vi "Create Framework.vi"(8 "error in (no error)":errorcluster, 11 "Application Data in":T1={"Item Tree Control"=refnum, "Top-Level VI"=refnum, "menu reference"=refnum, "queue"=refnum, "Stop Pointer"=refnum, "Buffer Variant"=variant, "server ID"=refnum, "framework tag"="", "Values"=refnum, "Hex"=refnum, "ASCII"=refnum, "lines visible"=0, "values padding"=0, "current buffer data"={"decimation"=0, "avg bandwidth"=0.0, "channels"=[], "byte order"=enum."little-endian", "buffer descriptor"={"buffer type"=enum."Engine", "plugin id"=0, "group id"=0, "transfer id"=0, "offset"=0, "length"=0}, "values channels"={"index"=0, "count"=0, "engine offset"=0}, "select start offset"=18446744073709551615, "select end offset"=0, "channel index"=-1}, "Framework Configuration"=refnum} {"current buffer data"."channels"."configuration"."string offset" format="%d bytes"; "current buffer data"."avg bandwidth" format="%.0g bytes"}) -> (0 "error out":errorcluster, 2 "framework tag":string, 3 "Application Data Out":T1={"Item Tree Control"=refnum, "Top-Level VI"=refnum, "menu reference"=refnum, "queue"=refnum, "Stop Pointer"=refnum, "Buffer Variant"=variant, "server ID"=refnum, "framework tag"="", "Values"=refnum, "Hex"=refnum, "ASCII"=refnum, "lines visible"=0, "values padding"=0, "current buffer data"={"decimation"=0, "avg bandwidth"=0.0, "channels"=[], "byte order"=enum."little-endian", "buffer descriptor"={"buffer type"=enum."Engine", "plugin id"=0, "group id"=0, "transfer id"=0, "offset"=0, "length"=0}, "values channels"={"index"=0, "count"=0, "engine offset"=0}, "select start offset"=18446744073709551615, "select end offset"=0, "channel index"=-1}, "Framework Configuration"=refnum} {"current buffer data"."channels"."configuration"."string offset" format="%d bytes"; "current buffer data"."avg bandwidth" format="%.0g bytes"})   [LabVIEW 2019, in "DSF Core.lvlib"]
uses:
  DSF Core.lvlib
  Main VI/Application Data.ctl
  <vilib>/NI/Memory Manager/Classes/Pointer/Pointer.lvclass
  Classes/Configuration/Core/Framework/Framework Configuration.lvclass
  Buffer Reader/Queue Data.ctl
  Buffer Reader/Buffer Data.ctl
  Classes/Configuration/Core/Transfer/Channel Configuration.ctl
  Typedefs/Core Channel Configuration.ctl
  Typedefs/DSF Data Type.ctl
  Typedefs/DSF Settings Info.ctl
  Typedefs/DSF Byte Order.ctl
  Classes/Thread/Data Server/DSF Buffer Subset Descriptor.ctl
  Typedefs/DSF Buffer Type.ctl
  Main VI/Values Channels.ctl
  ID to Tree Items/Tree Item Type.ctl
  Classes/Configuration/Core/Channel/Channel Configuration.lvclass
  Classes/Configuration/Core/Transfer/Transfer Configuration.lvclass
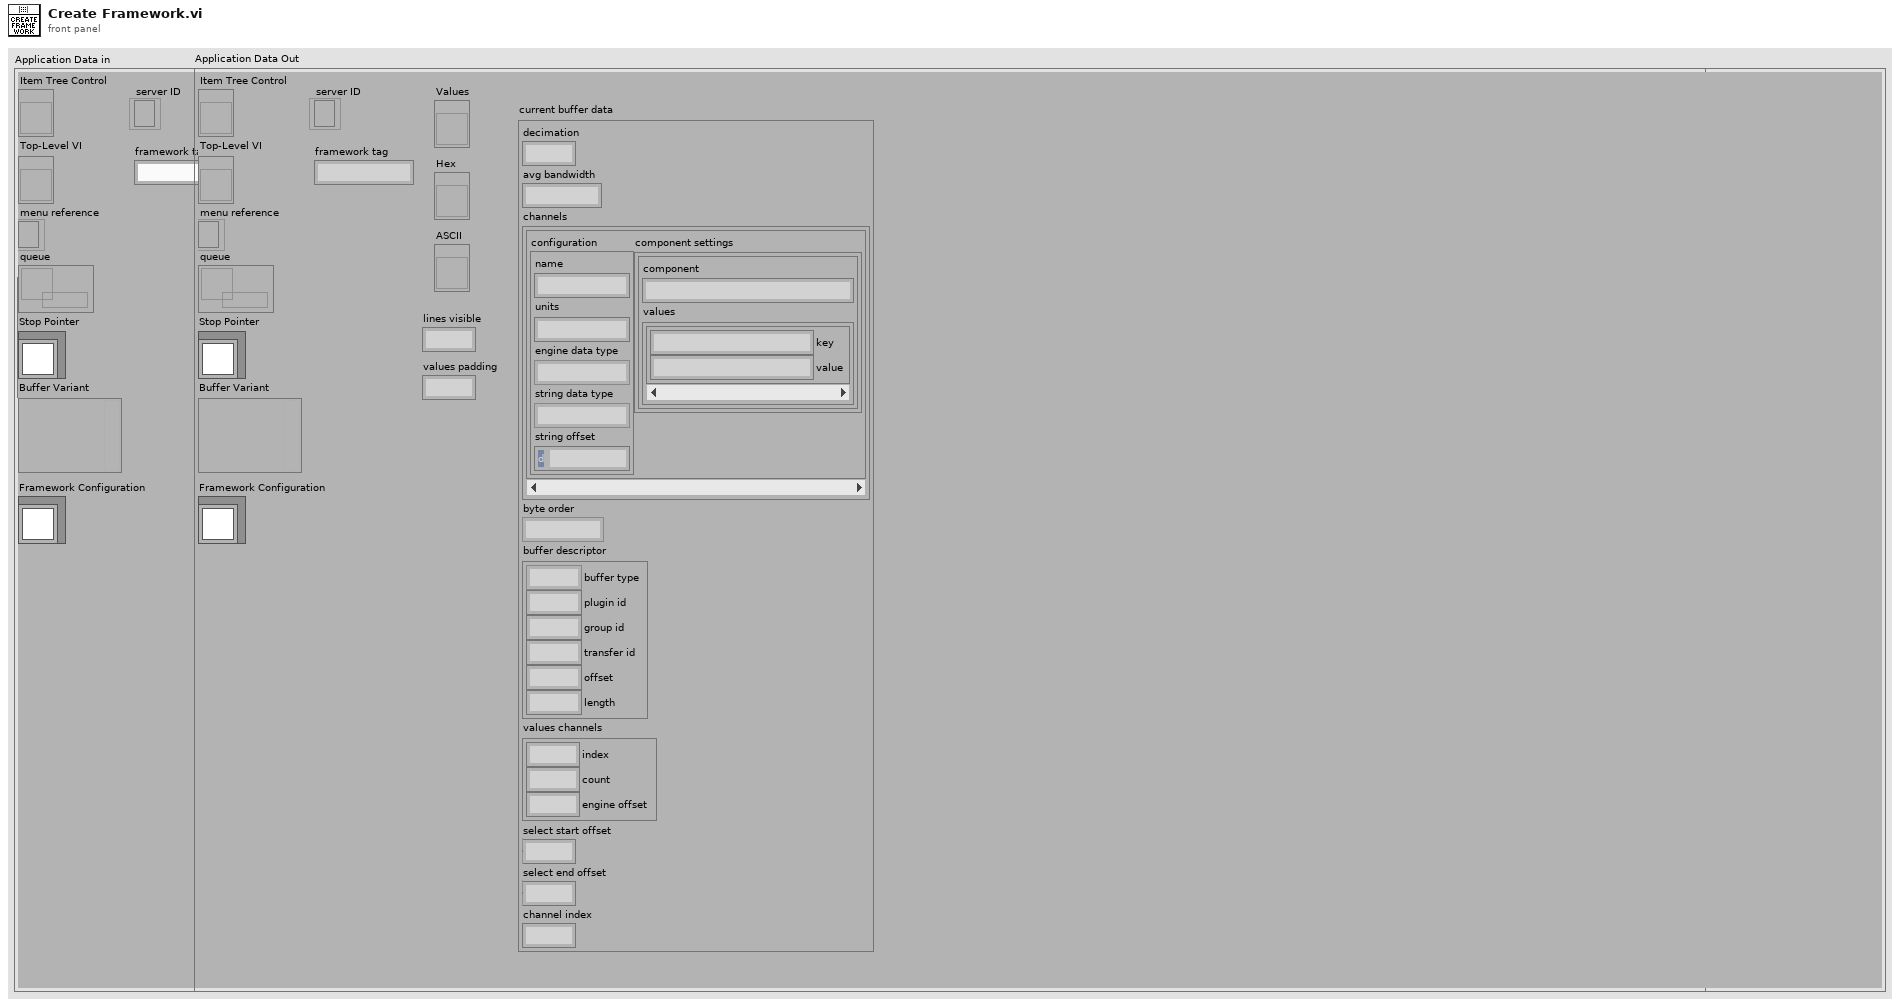
[diagram p1: front panel]
types:
  T1 = typedef "DSF Core.lvlib/Application Data.ctl" = cluster{"Item Tree Control":refnum<vi>, "Top-Level VI":refnum<vi>, "menu reference":refnum<k9>, "queue":refnum<queue>, "Stop Pointer":refnum<class "Pointer.lvclass">, "Buffer Variant":variant, "server ID":refnum<k5>, "framework tag":string, "Values":refnum<vi>, "Hex":refnum<vi>, "ASCII":refnum<vi>, "lines visible":i32, "values padding":i32, "current buffer data":T2, "Framework Configuration":refnum<class "Framework Configuration.lvclass">}
  T2 = typedef "DSF Core.lvlib/Buffer Data.ctl" = cluster{"decimation":u64, "avg bandwidth":dbl, "channels":T3[], "byte order":T7, "buffer descriptor":T8, "values channels":T10, "select start offset":u64, "select end offset":u64, "channel index":i32}
  T3 = typedef "DSF Core.lvlib/Transfer Configuration.lvclass/Channel Configuration.ctl" = cluster{"configuration":T4, "component settings":T6[]}
  T4 = typedef "DSF Core.lvlib/Channel Configuration.lvclass/Core Channel Configuration.ctl" = cluster{"name":string, "units":string, "engine data type":T5, "string data type":T5, "string offset":u64}
  T5 = typedef "DSF Core.lvlib/DSF Data Type.ctl" = enum8{"Bool", "SGL", "DBL", "I8", "I16", "I32", "I64", "U8", "U16", "U32", "U64"}
  T6 = typedef "DSF Core.lvlib/DSF Settings Info.ctl" = cluster{"component":string, "values":cluster{"key":string, "value":string}[]}
  T7 = typedef "DSF Core.lvlib/DSF Byte Order.ctl" = enum8{"big-endian", "little-endian"}
  T8 = typedef "DSF Core.lvlib/DSF Buffer Subset Descriptor.ctl" = cluster{"buffer type":T9, "plugin id":i32, "group id":i32, "transfer id":i32, "offset":u64, "length":i64}
  T9 = typedef "DSF Core.lvlib/DSF Buffer Type.ctl" = enum16{"Engine", "String"}
  T10 = typedef "DSF Core.lvlib/Values Channels.ctl" = cluster{"index":i32, "count":i32, "engine offset":u64}
  T11 = typedef "DSF Core.lvlib/Tree Item Type.ctl" = enum16{"Framework", "Plugin Group", "Plugin", "Group", "Transfer", "Buffer", "Channel"}
  T12 = typedef "DSF Core.lvlib/Tree Item.ctl" = cluster{"Left Cell String":string, "Child Text":string[], "Child Tag":string, "Glyph Index":i32}
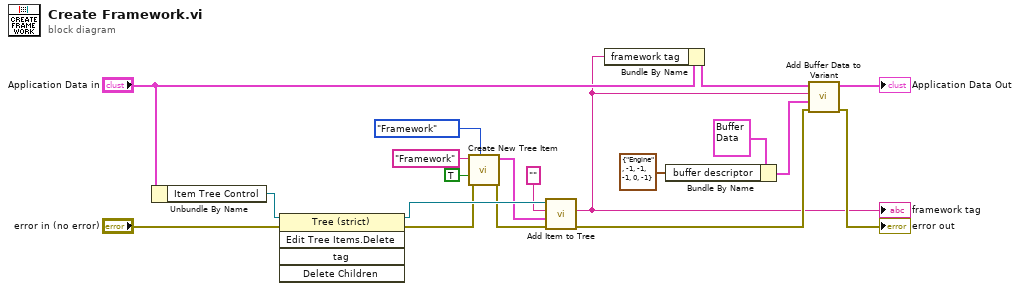
[diagram p0: block diagram]
diagram:
  n1 = Unbundle By Name("Application Data in") -> ("Item Tree Control"=w12:refnum<vi>)
  n2 = invoke class="Tree (strict)" method="Edit Tree Items.Delete"(reference=w12, error in="error in (no error)") -> (reference out=w19:refnum<vi>, error out=w18:errorcluster)  [unwired: 3 in, 3 out]
  n3 = call "Create New Tree Item.vi"("Item Type"=Tree_Item_Type."Framework", "error in"=w18, "found?"=TRUE, "Left Cell String"="Framework") -> ("error out"=w17:errorcluster, "Item"=w16:T12)  [unwired: 6 in]
  n4 = call "Add Item to Tree.vi"("error in (no error)"=w17, "Item"=w16, "parent tag"="", "TreeControl in"=w19) -> ("error out"=w9:errorcluster, "new item tag"=w1:string)  [unwired: 5 in, 1 out]
  "framework tag" <- w1
  n5 = Bundle By Name(cluster="Application Data in", "framework tag"=w1) -> (w2:T1)
  n6 = Bundle By Name(cluster=T2 {"decimation"=0, "avg bandwidth"=0.0, "channels"=[], "byte order"=enum."big-endian", "buffer descriptor"={"buffer type"=enum."Engine", "plugin id"=0, "group id"=0, "transfer id"=0, "offset"=0, "length"=0}, "values channels"={"index"=0, "count"=0, "engine offset"=0}, "select start offset"=18446744073709551615, "select end offset"=0, "channel index"=-1} ("Buffer data"), "buffer descriptor"=T8 {"buffer type"=enum."Engine", "plugin id"=-1, "group id"=-1, "transfer id"=-1, "offset"=0, "length"=-1}) -> (w6:T2)
  n7 = call "Add Buffer Data to Variant.vi"("error in (no error)"=w9, "Buffer data"=w6, "tag"=w1, "Application Data In in"=w2) -> ("error out"=→"error out":errorcluster, "Application Data In out"=→"Application Data Out":T1)  [unwired: 6 in]
